vi "Calibracao.vi"() -> ()   [LabVIEW 2019]
uses:
  <vilib>/Utility/config.llb/Config Data RefNum.ctl
  padrao_array_cluster_calibracao.ctl
  <vilib>/Utility/config.llb/Write Key (String).vi
  <vilib>/Utility/config.llb/Write Key (Double).vi
  <vilib>/Utility/config.llb/Read Key (String).vi
  <vilib>/Utility/config.llb/Read Key (Double).vi
  <vilib>/Utility/config.llb/NI_LVConfig.lvlib
panel:
  in  "Search Button":bool
  in  "barra_de_pesquisa":string
  out "Instrumentos nao modificados":T1
  in  "Instrumentos":T1
  out "Status":string
  in  "Remove Button":bool
  in  "Cancelar Modificacao":bool
  out "error out":errorcluster
  out "refnum out":T2
  in  "Salvar":bool
  in  "[ESC]":bool
  # "CALIBRA敲O"
  # "Digite no campo de busca a TAG desejada:"
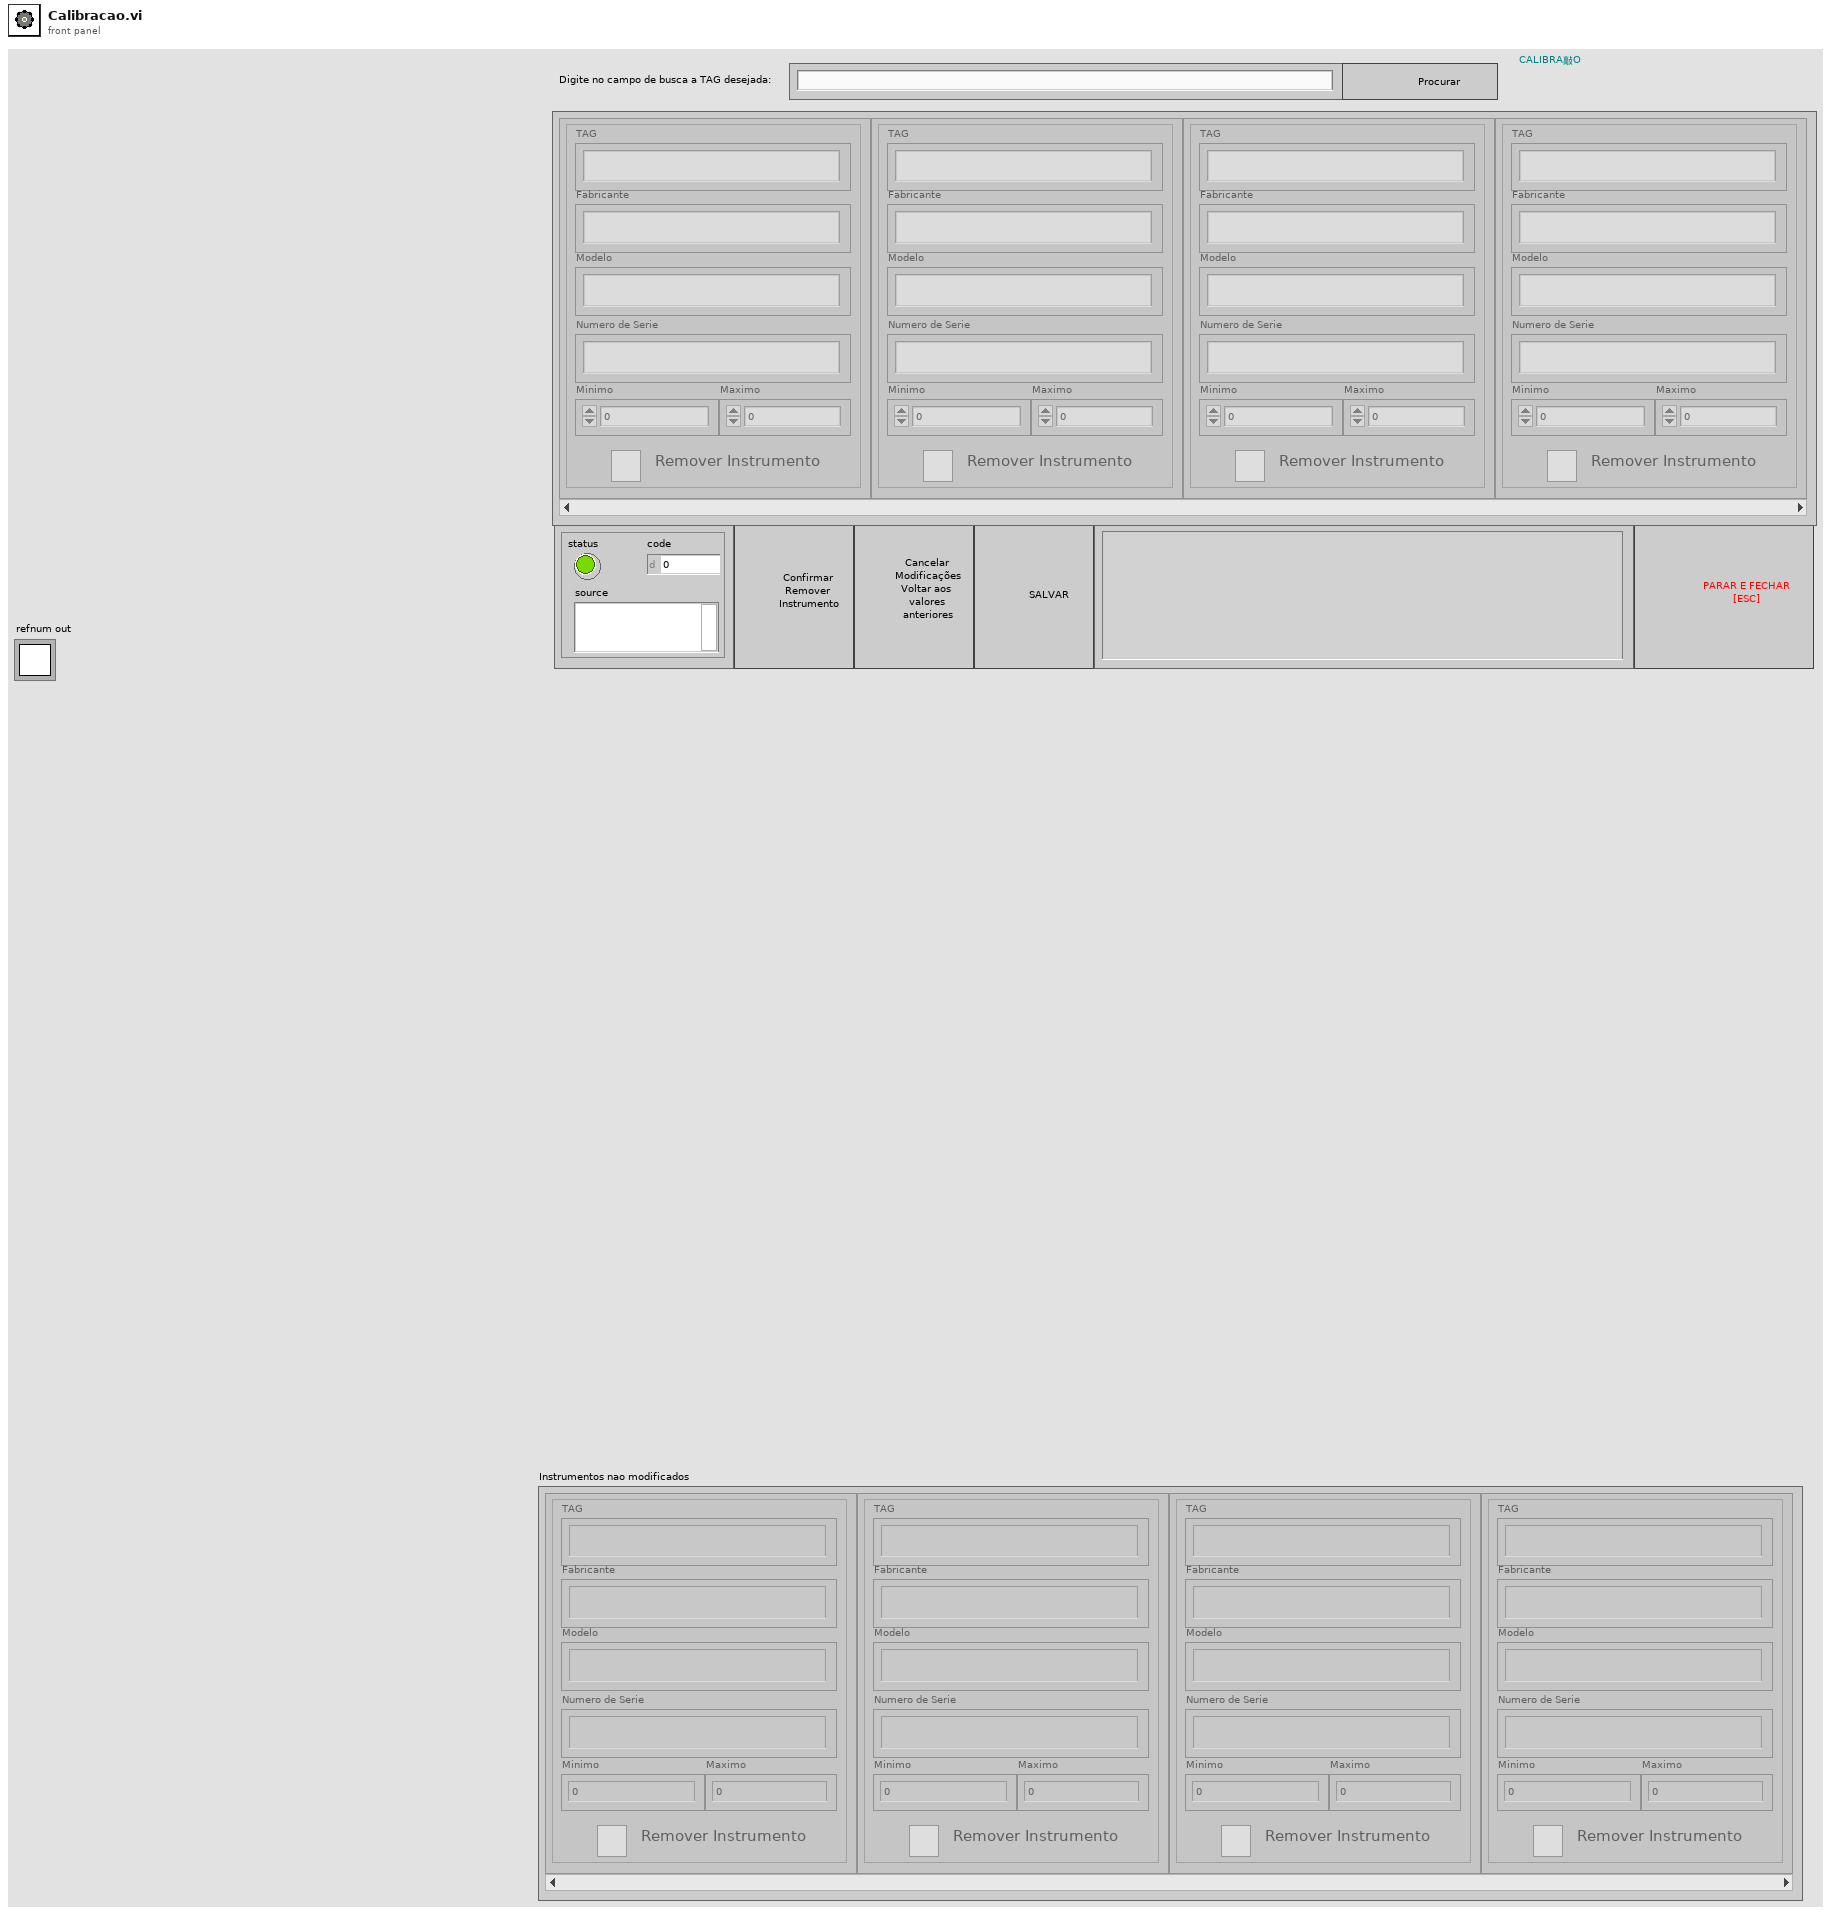
[diagram p1: front panel]
types:
  T1 = typedef "padrao_array_cluster_calibracao.ctl" = cluster{"TAG":string, "Minimo":dbl, "Fabricante":string, "Maximo":dbl, "remover_dipositvo":bool, "Modelo":string, "Numero de Serie":string}[]
  T2 = typedef "NI_LVConfig.lvlib/Config Data RefNum.ctl" = refnum<k1>
  T3 = enum8{"Enabled", "Disabled", "Disabled and Grayed Out"}
  T4 = cluster{"TAG":string, "Minimo":dbl, "Fabricante":string, "Maximo":dbl, "remover_dipositvo":bool, "Modelo":string, "Numero de Serie":string}
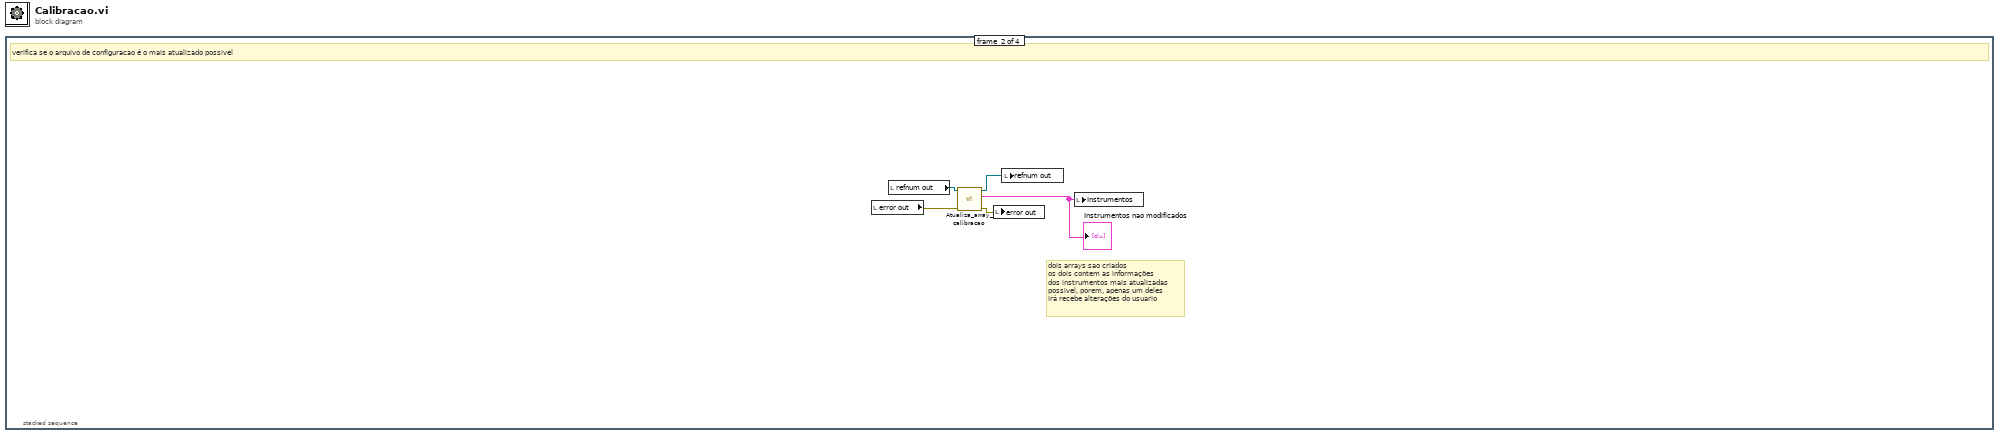
[diagram p0: block diagram]
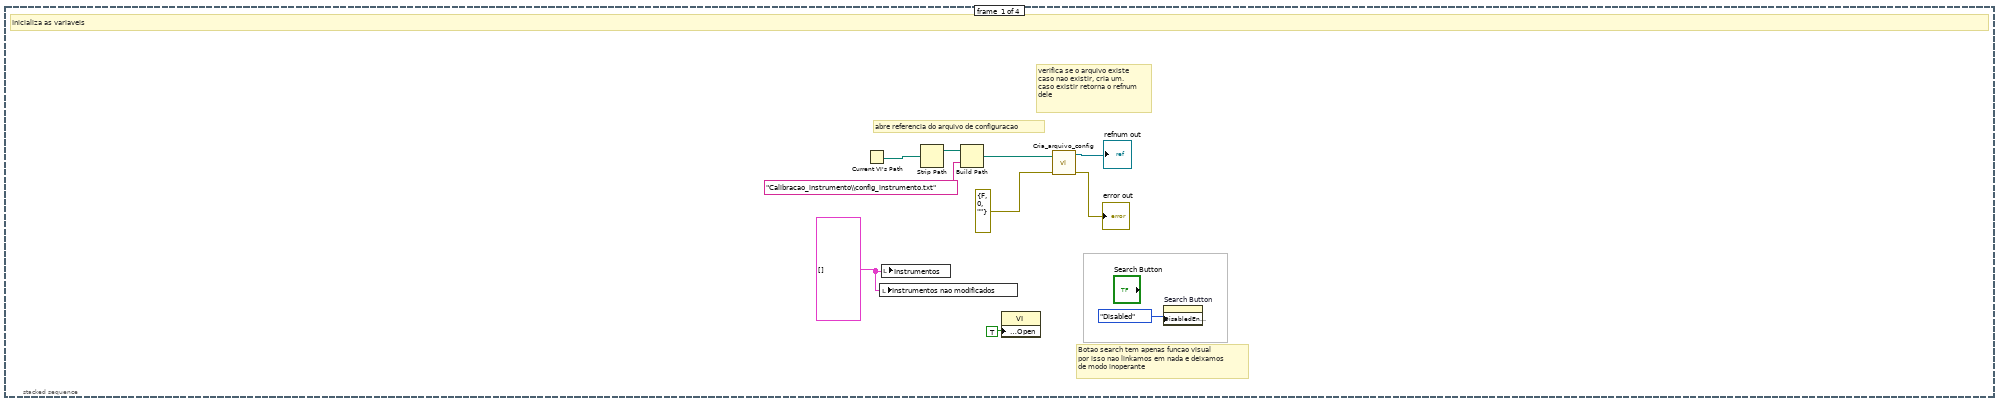
[diagram p2: hidden frame]
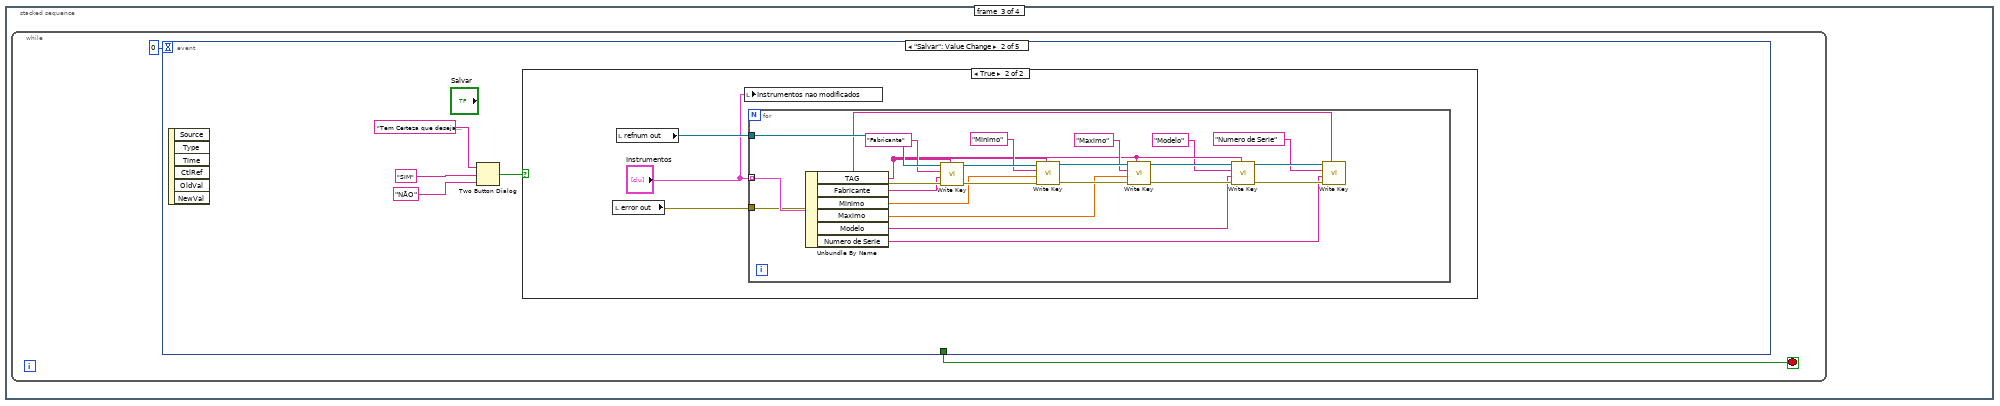
[diagram p3: hidden frame]
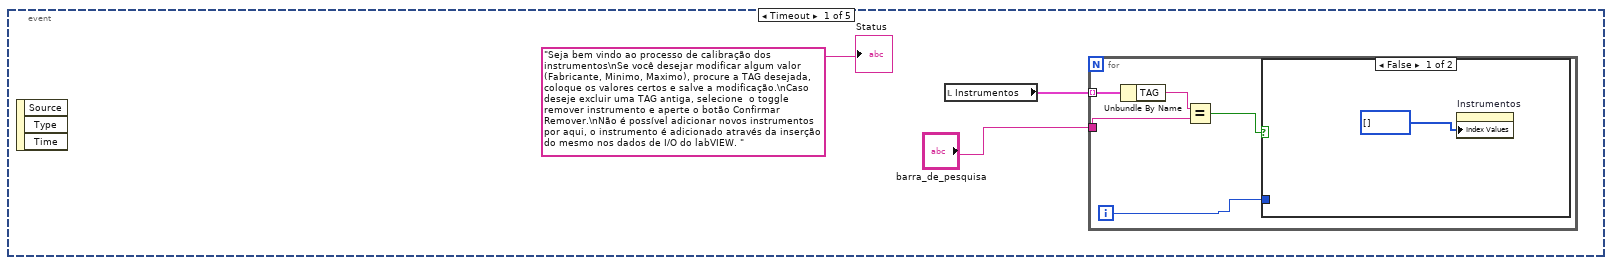
[diagram p4: hidden frame]
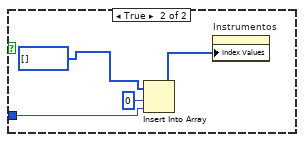
[diagram p5: hidden frame]
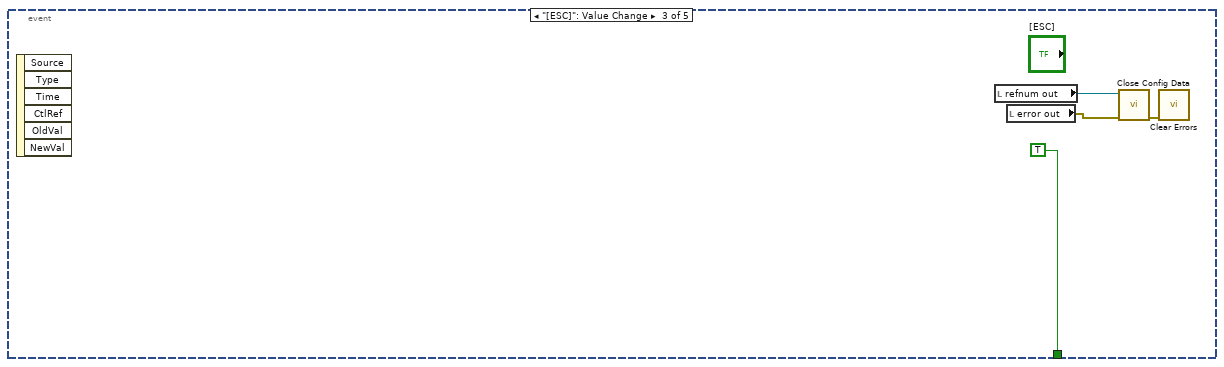
[diagram p7: hidden frame]
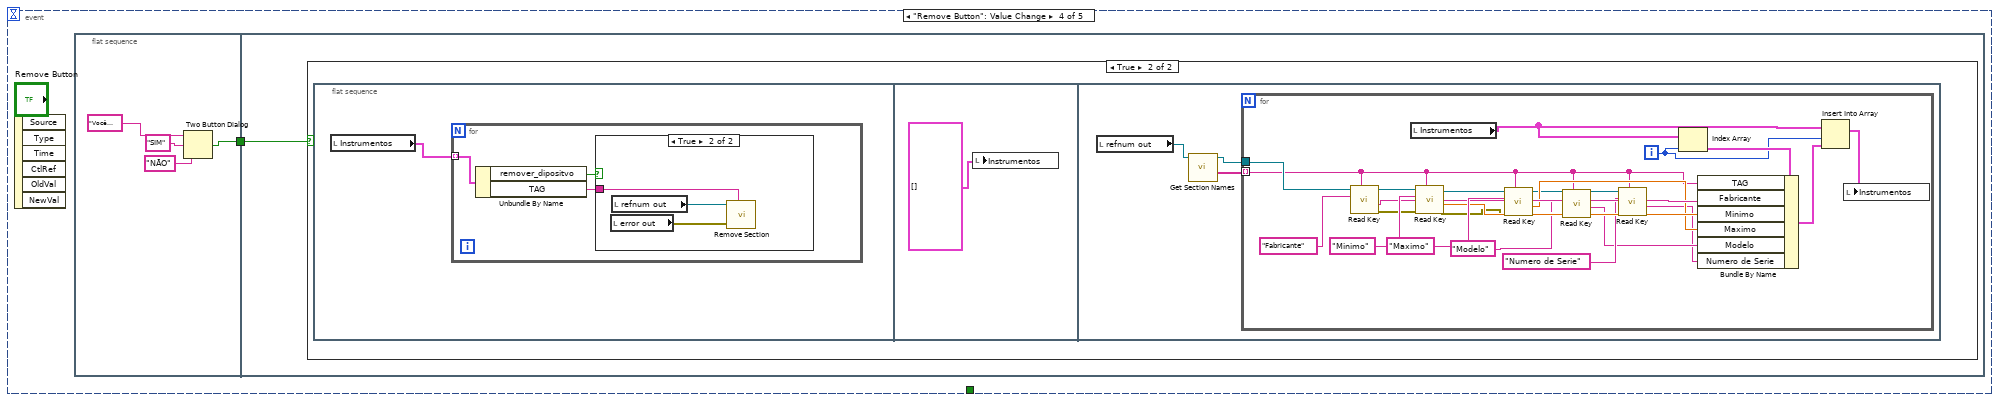
[diagram p8: hidden frame]
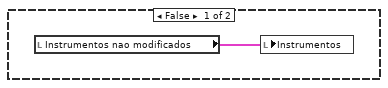
[diagram p9: hidden frame]
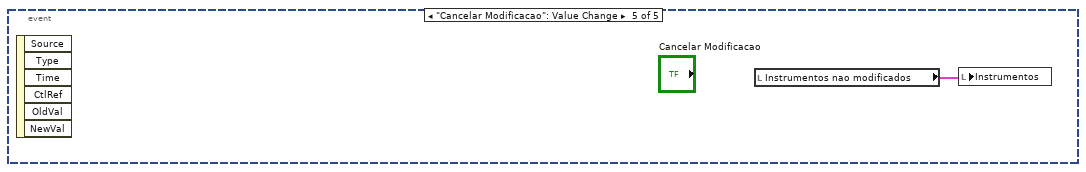
[diagram p11: hidden frame]
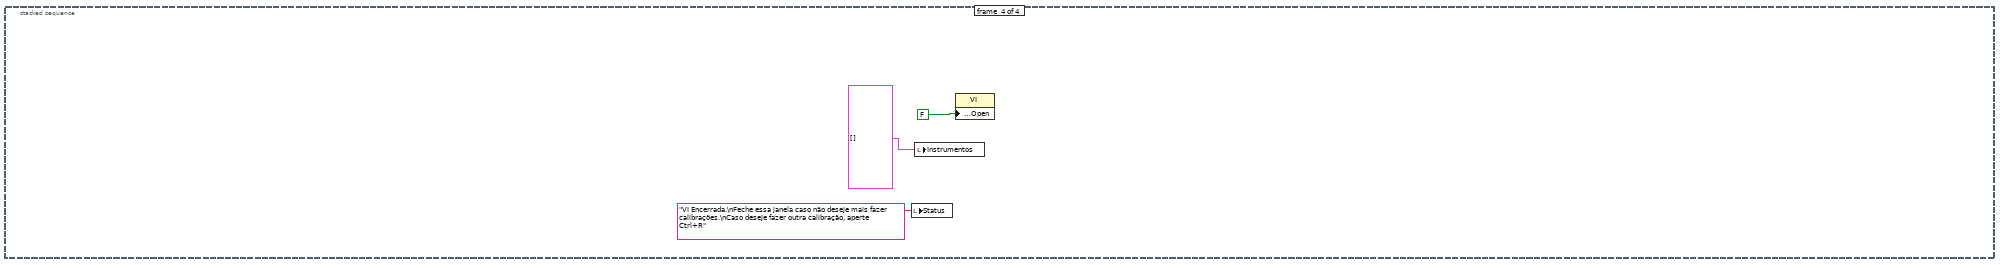
[diagram p12: hidden frame]
diagram:
  n1 = stacked-sequence {
    frame #0 {
      w6 = T1 [] ("Instrumentos")
      # "Botao search tem apenas funcao visual\npor isso nao linkamos em nada e deixamos\nde modo inoperante"
      # "verifica se o arquivo existe \ncaso nao existir, cria um.\ncaso existir retorna o refnum\ndele"
      # "abre referencia do arquivo de configuracao"
      # "Inicializa as variaveis"
      n2 = Current VI's Path() -> (path=w7:path)
      n3 = local write "Instrumentos nao modificados"(w6) -> ()
      n4 = local write "Instrumentos"(w6) -> ()
      n5 = Strip Path(path=w7) -> (stripped path=w9:path)  [unwired: 1 out]
      n6 = Build Path(base path=w9, name or relative path="Calibracao_instrumento\\config_instrumento.txt") -> (appended path=w5:path)
      n7 = property class="VI"("Front Panel.Open"=TRUE ("Front Panel Window:Open")) -> ()  [unwired: 2 in, 2 out]
      n8 = call "Cria_arquivo_config.vi"("error in (no error)"=errorcluster {"status"=FALSE, "code"=0, "source"=""}, "refnum in"=w5) -> ("error out"=→"error out":errorcluster, "refnum"=→"refnum out":T2)  [unwired: 8 in]
      n9 = property on="Search Button" class="Bool"("DisabledEnum"=T3."Disabled" ("Disabled")) -> ()  [unwired: 2 in, 2 out]
    }
    frame #1 {
      # "dois arrays sao criados\nos dois contem as informações \ndos instrumentos mais atualizadas\npossivel, porem, apenas um deles \nirá recebe alterações do usuario"
      # "verifica se o arquivo de configuracao é o mais atualizado possivel"
      n10 = local read "error out"() -> (w14:errorcluster)
      n11 = local read "refnum out"() -> (w15:T2)
      n12 = call "Atualiza_array_calibracao.vi"("error in (no error)"=w14, "refnum"=w15) -> ("error out"=w12:errorcluster, "Instrumentos"=w11:T1, "refnum out"=w13:T2)  [unwired: 7 in]
      "Instrumentos nao modificados" <- w11
      n13 = local write "error out"(w12) -> ()
      n14 = local write "refnum out"(w13) -> ()
      n15 = local write "Instrumentos"(w11) -> ()
    }
    frame #2 {
      n16 = while {
        stop <- w17 stop-if-true
        n17 = event shown="[1] \"Salvar\": Value Change" {
          selector: _ -> [_ _ _ _ _]
          dyn-events: _ -> [_ _ _ _ _]
          timeout: 0 -> [_ _ _ _ _]
          tunnel: [_ _ TRUE _ _] -> w17
          event Timeout {
            n18 = event-data() -> ()  [unwired: 1 in, 3 out]
            n19 = local read "Instrumentos"() -> (w19:T1)
            n20 = for {
              tunnel: w19 -> [w25] mode=indexing
              tunnel: "barra_de_pesquisa" -> [w23]
              i -> [w22]
              n21 = Unbundle By Name(w25) -> ("TAG"=w24:string)
              n22 = Equal?(x=w24, y=w23) -> (x = y?=w21:bool)
              n23 = case shown="False" w21 {
                tunnel: w22 -> [_ w29]
                frame False {
                  n24 = property on="Instrumentos" class="Arr (strict)"("Index Values"=u32[] []) -> ()  [unwired: 2 in, 2 out]
                }
                frame True {
                  n25 = Insert Into Array(array=u32[] [] ("Index Values"), index=0, new element=w29) -> (w27:u32[])
                  n26 = property on="Instrumentos" class="Arr (strict)"("Index Values"=w27) -> ()  [unwired: 2 in, 2 out]
                }
              }
            }
            "Status" <- "Seja bem vindo ao processo de calibração dos instrumentos\nSe você desejar modificar algum valor (Fabricante, Minimo, Maximo), procure a TAG desejada, coloque os valores certos e salve a modificação.\nCaso deseje excluir uma TAG antiga, selecione  o toggle remover instrumento e aperte o botão Confirmar Remover.\nNão é possível adicionar novos instrumentos por aqui, o instrumento é adicionado através da inserção do mesmo nos dados de I/O do labVIEW. " ("Status")
          }
          event "Salvar": Value Change {
            n27 = event-data() -> ()  [unwired: 1 in, 6 out]
            n28 = Two Button Dialog(message="Tem Certeza que deseja salvar as alterações Feitas?\nOs valores antigos serão perdidos e não poderão ser recuperados", 1:"NÃO" ("F button name (\"Cancel\")"), 2:"SIM" ("T button name (\"OK\")")) -> (T button?=w34:bool)
            n29 = case shown="True" w34 {
              frame False {
              }
              frame True {
                n30 = local read "error out"() -> (w36:errorcluster)
                n31 = local read "refnum out"() -> (w37:T2)
                n32 = local write "Instrumentos nao modificados"("Instrumentos") -> ()
                n33 = for {
                  tunnel: "Instrumentos" -> [w59] mode=indexing
                  tunnel: w37 -> [w55]
                  tunnel: w36 -> [w58]
                  n34 = Unbundle By Name(w59) -> ("TAG"=w42:string, "Fabricante"=w49:string, "Minimo"=w48:dbl, "Maximo"=w47:dbl, "Modelo"=w39:string, "Numero de Serie"=w38:string)
                  n35 = call-poly <vilib>:"Write Key.vi"("section"=w42, "error in (no error)"=w58, "value"=w49, "key"="Fabricante", "refnum"=w55) -> ("error out"=w57:errorcluster, "refnum out"=w54:T2)  [unwired: 4 in, 1 out]
                  n36 = call-poly <vilib>:"Write Key.vi"("section"=w42, "error in (no error)"=w57, "value"=w48, "key"="Minimo", "refnum"=w54) -> ("error out"=w56:errorcluster, "refnum out"=w53:T2)  [unwired: 4 in, 1 out]
                  n37 = call-poly <vilib>:"Write Key.vi"("section"=w42, "error in (no error)"=w56, "value"=w47, "key"="Maximo", "refnum"=w53) -> ("error out"=w43:errorcluster, "refnum out"=w45:T2)  [unwired: 4 in, 1 out]
                  n38 = call-poly <vilib>:"Write Key.vi"("section"=w42, "error in (no error)"=w43, "value"=w39, "key"="Modelo", "refnum"=w45) -> ("error out"=w46:errorcluster, "refnum out"=w44:T2)  [unwired: 4 in, 1 out]
                  n39 = call-poly <vilib>:"Write Key.vi"("section"=w42, "error in (no error)"=w46, "value"=w38, "key"="Numero de Serie", "refnum"=w44) -> ()  [unwired: 4 in, 3 out]
                }
              }
            }
          }
          event "[ESC]": Value Change {
            n40 = event-data() -> ()  [unwired: 1 in, 6 out]
            n41 = local read "refnum out"() -> (w62:T2)
            n42 = local read "error out"() -> (w60:errorcluster)
            n43 = call <vilib>:"Close Config Data.vi"("error in (no error)"=w60, "refnum"=w62) -> ("error out"=w61:errorcluster)  [unwired: 8 in, 1 out]
            n44 = call <vilib>:"Clear Errors.vi"("error in (no error)"=w61) -> ()  [unwired: 5 in, 2 out]
          }
          event "Remove Button": Value Change {
            n45 = event-data() -> ()  [unwired: 1 in, 6 out]
            n46 = flat-sequence {
              tunnel: [w65] -> w64
              tunnel: w64 -> [w69]
              frame #0 {
                n47 = Two Button Dialog(message="Você Clicou Para remover os instrumentos selecioandos.\nVocê tem certeza que deseja removê-los?", 1:"NÃO" ("F button name (\"Cancel\")"), 2:"SIM" ("T button name (\"OK\")")) -> (T button?=w65:bool)
              }
              frame #1 {
                n48 = case shown="True" w69 {
                  frame False {
                    n49 = local read "Instrumentos nao modificados"() -> (w70:T1)
                    n50 = local write "Instrumentos"(w70) -> ()
                  }
                  frame True {
                    n51 = flat-sequence {
                      frame #0 {
                        n52 = local read "Instrumentos"() -> (w71:T1)
                        n53 = for {
                          tunnel: w71 -> [w74] mode=indexing
                          n54 = Unbundle By Name(w74) -> ("remover_dipositvo"=w73:bool, "TAG"=w72:string)
                          n55 = case shown="True" w73 {
                            tunnel: w72 -> [_ w77]
                            frame False {
                            }
                            frame True {
                              n56 = local read "error out"() -> (w75:errorcluster)
                              n57 = local read "refnum out"() -> (w76:T2)
                              n58 = call <vilib>:"Remove Section.vi"("section"=w77, "error in (no error)"=w75, "refnum"=w76) -> ()  [unwired: 6 in, 3 out]
                            }
                          }
                        }
                      }
                      frame #1 {
                        n59 = local write "Instrumentos"(T1 [] ("Instrumentos")) -> ()
                      }
                      frame #2 {
                        n60 = local read "refnum out"() -> (w79:T2)
                        n61 = call <vilib>:"Get Section Names.vi"("refnum"=w79) -> ("section names"=w80:string[], "refnum out"=w81:T2)  [unwired: 8 in, 1 out]
                        n62 = for {
                          tunnel: w80 -> [w85] mode=indexing
                          tunnel: w81 -> [w105]
                          i -> [w97]
                          n63 = call-poly <vilib>:"Read Key.vi"("section"=w85, "key"="Fabricante", "refnum"=w105) -> ("error out"=w94:errorcluster, "value"=w100:string, "refnum out"=w95:T2)  [unwired: 5 in, 1 out]
                          n64 = local read "Instrumentos"() -> (w93:T1)
                          n65 = call-poly <vilib>:"Read Key.vi"("section"=w85, "error in (no error)"=w94, "key"="Minimo", "refnum"=w95) -> ("error out"=w86:errorcluster, "value"=w99:dbl, "refnum out"=w101:T2)  [unwired: 4 in, 1 out]
                          n66 = call-poly <vilib>:"Read Key.vi"("section"=w85, "error in (no error)"=w86, "key"="Maximo", "refnum"=w101) -> ("error out"=w91:errorcluster, "value"=w90:dbl, "refnum out"=w89:T2)  [unwired: 4 in, 1 out]
                          n67 = call-poly <vilib>:"Read Key.vi"("section"=w85, "error in (no error)"=w91, "key"="Modelo", "refnum"=w89) -> ("error out"=w87:errorcluster, "value"=w83:string, "refnum out"=w88:T2)  [unwired: 4 in, 1 out]
                          n68 = call-poly <vilib>:"Read Key.vi"("section"=w85, "error in (no error)"=w87, "key"="Numero de Serie", "refnum"=w88) -> ("value"=w82:string)  [unwired: 4 in, 3 out]
                          n69 = Index Array(array=w93, index=w97) -> (element=w106:T4)
                          n70 = Bundle By Name(cluster=w106, "TAG"=w85, "Fabricante"=w100, "Minimo"=w99, "Maximo"=w90, "Modelo"=w83, "Numero de Serie"=w82) -> (w98:T4)
                          n71 = Insert Into Array(array=w93, index=w97, new element=w98) -> (w96:T1)
                          n72 = local write "Instrumentos"(w96) -> ()
                        }
                      }
                    }
                  }
                }
              }
            }
          }
          event "Cancelar Modificacao": Value Change {
            n73 = event-data() -> ()  [unwired: 1 in, 6 out]
            n74 = local read "Instrumentos nao modificados"() -> (w107:T1)
            n75 = local write "Instrumentos"(w107) -> ()
          }
        }
      }
    }
    frame #3 {
      n76 = local write "Status"("VI Encerrada.\nFeche essa janela caso não deseje mais fazer calibrações.\nCaso deseje fazer outra calibração, aperte Ctrl+R" ("Status")) -> ()
      n77 = local write "Instrumentos"(T1 [] ("Instrumentos")) -> ()
      n78 = property class="VI"("Front Panel.Open"=FALSE ("Front Panel Window:Open")) -> ()  [unwired: 2 in, 2 out]
    }
  }
